vi "add_sync.vi"(8 "error in (no error)":errorcluster, 10 "Sync Words":i8[](array[numeric]), 11 "Payload Bits":i8[](array[numeric]) caption="Payload") -> (0 "error out":errorcluster caption="error in (no error)", 3 "Transmitted Sequence":i8[](array[numeric]) caption="Key Bit Sequence")   [LabVIEW 2012]
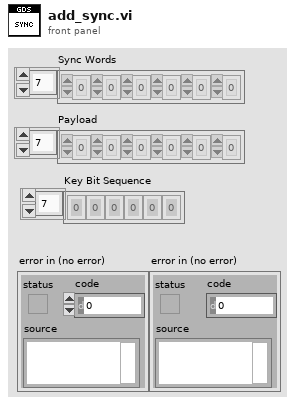
[diagram p1: front panel]
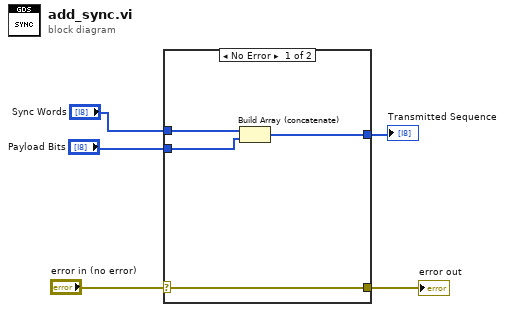
[diagram p0: block diagram]
diagram:
  n1 = case shown="No Error" "error in (no error)" {
    selector: "error in (no error)" -> [w9 w10]
    tunnel: [w9 w10] -> w4
    tunnel: "Payload Bits" -> [w7 _]
    tunnel: "Sync Words" -> [w8 _]
    tunnel: [w6 _] -> w1
    frame No Error {
      n2 = Build Array (concatenate)(w8, w7) -> (w6:i8[])
    }
    frame Error {
    }
  }
  "Transmitted Sequence" <- w1
  "error out" <- w4
